vi "AnalogOutput.vi"() -> ()   [LabVIEW 2012]
panel:
  out "peak-peak":dbl format="%#_6p"
  out "+peak":dbl format="%#_6p"
  in  "stop":bool
  out "dc":dbl format="%#.6p"
  out "Waveform Graph":cluster{"x0":dbl, "dx":dbl, "magnitude":dbl[]}(graph)
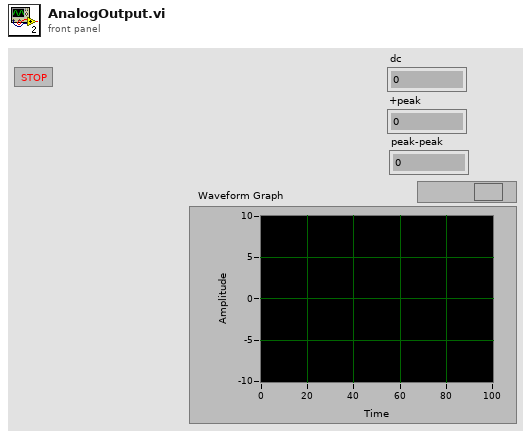
[diagram p1: front panel]
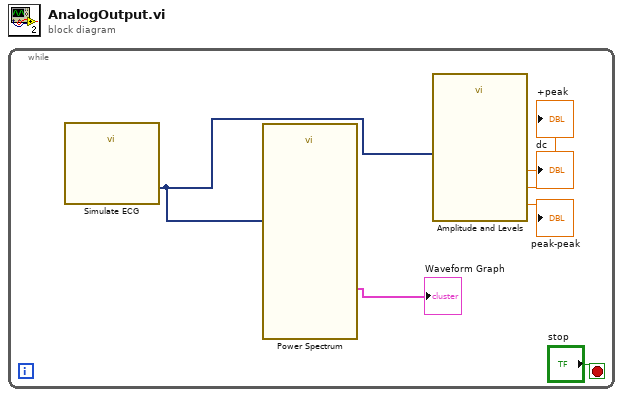
[diagram p0: block diagram]
diagram:
  n1 = while {
    stop <- "stop" stop-if-true
    n2 = call "Simulate ECG"() -> ("ECG"=w1:dynamicdata)  [unwired: 10 in, 1 out]
    n3 = call "Power Spectrum"("input signal"=w1) -> ("spectrum"=→"Waveform Graph":cluster{"x0":dbl, "dx":dbl, "magnitude":dbl[]})  [unwired: 13 in, 5 out]
    n4 = call "Amplitude and Levels"("input signal"=w1) -> ("dc"=→"dc":dbl, "+peak"=→"+peak":dbl, "peak-peak"=→"peak-peak":dbl)  [unwired: 15 in, 1 out]
  }
